vi "OE1022D_Close.vi"(2 "错误输入（无错误）":errorcluster, 3 "VISA resource name":refnum<visa-resource-name>) -> (0 "错误输出":errorcluster)   [LabVIEW 2019]
doc: "Configures the reference source and the internal oscillator."
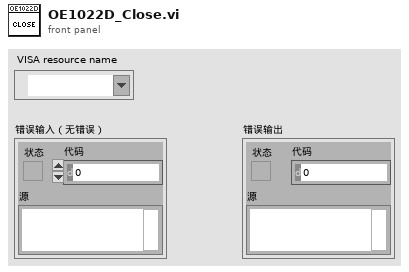
[diagram p1: front panel]
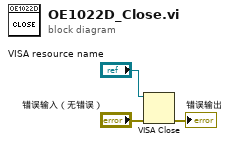
[diagram p0: block diagram]
diagram:
  n1 = VISA Close(VISA resource name="VISA resource name", error in (no error)="错误输入（无错误）") -> (error out=→"错误输出":errorcluster)
